vi "BRig_RT__Case_Exp__State_TimeoutPre.vi"(6 "input_dataExp":u16[](array[numeric]), 9 "input_dataBlock":u16[][](array[numeric]), 11 "input_dataCurrent":u16[](array[numeric])) -> (1 "output_dataBlock":u16[][](array[numeric]), 3 "output_dataCurrent":u16[](array[numeric]))   [LabVIEW 2014]
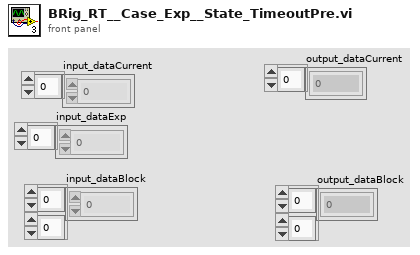
[diagram p1: front panel]
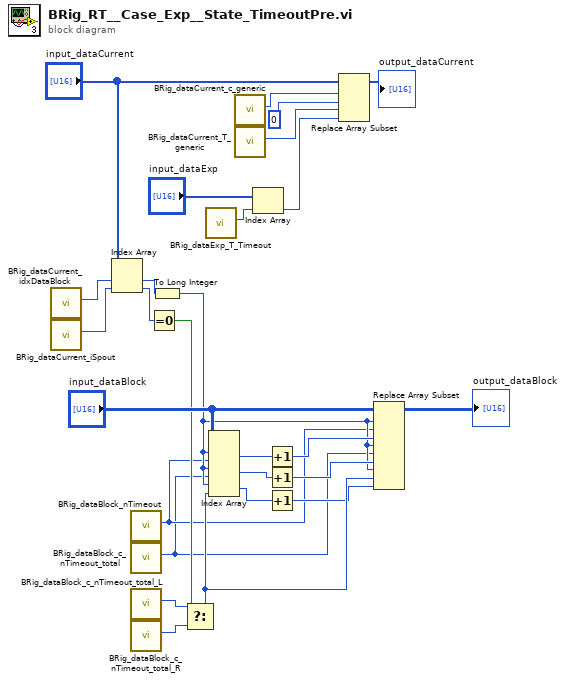
[diagram p0: block diagram]
diagram:
  n1 = call "BRig_dataCurrent_idxDataBlock.vi"() -> ("output_idxDataBlock"=w20:i32)  [unwired: 11 in]
  n2 = call "BRig_dataCurrent_iSpout.vi"() -> ("output_iSpout"=w18:i32)  [unwired: 11 in]
  n3 = Index Array(array="input_dataCurrent", index #1=w20, index #2=w18) -> (element #1=w19:u16, element #2=w17:u16)
  n4 = call "BRig_dataBlock_nTimeout.vi"() -> ("output_nTimeout"=w4:i32)  [unwired: 11 in]
  n5 = call "BRig_dataBlock_c_nTimeout_total.vi"() -> ("output_c_nTimeout_total"=w3:i32)  [unwired: 11 in]
  n6 = call "BRig_dataBlock_c_nTimeout_total_L.vi"() -> ("output_c_nTimeout_total_L"=w2:i32)  [unwired: 11 in]
  n7 = call "BRig_dataBlock_c_nTimeout_total_R.vi"() -> ("output_c_nTimeout_total_R"=w1:i32)  [unwired: 11 in]
  n8 = Equal To 0?(x=w17) -> (x = 0?=w6:bool)
  n9 = To Long Integer(number=w19) -> (32bit integer=w7:i32)
  n10 = Select(t=w2, s=w6, f=w1) -> (s? t:f=w11:i32)
  n11 = call "BRig_dataExp_T_Timeout.vi"() -> ("output_T_Timeout"=w21:i32)  [unwired: 11 in]
  n12 = Index Array(array="input_dataBlock", index (row) #1=w7, index (col) #1=w4, index (row) #2=w7, index (col) #2=w3, index (row) #3=w7, index (col) #3=w11) -> (element #1=w16:u16, element #2=w14:u16, element #3=w12:u16)
  n13 = call "BRig_dataCurrent_c_generic.vi"() -> ("output_count_generic"=w26:i32)  [unwired: 11 in]
  n14 = call "BRig_dataCurrent_T_generic.vi"() -> ("output_T_generic"=w25:i32)  [unwired: 11 in]
  n15 = Index Array(array="input_dataExp", index=w21) -> (element=w22:u16)
  n16 = Increment(x=w16) -> (x+1=w15:u16)
  n17 = Increment(x=w14) -> (x+1=w13:u16)
  n18 = Increment(x=w12) -> (x+1=w10:u16)
  n19 = Replace Array Subset(array="input_dataCurrent", new element #1=u16 0 ("new element/subarray"), index #1=w26, new element #2=w22, index #2=w25) -> (→"output_dataCurrent":u16[])
  n20 = Replace Array Subset(array="input_dataBlock", new element #1=w15, index (row) #1=w7, index (col) #1=w4, new element #2=w13, index (row) #2=w7, index (col) #2=w3, new element #3=w10, index (row) #3=w7, index (col) #3=w11) -> (→"output_dataBlock":u16[][])
